vi "Mock Launch Helper Loop.vi"(8 "error in (no error)":errorcluster, 11 "Mock Process in":refnum<class "Mock Process.lvclass">) -> (0 "error out":errorcluster, 3 "Mock Process out":refnum<class "Mock Process.lvclass">)   [LabVIEW 2020, in "Mock Process.lvclass"]
uses:
  Mock Process.lvclass
  C:/Git/astemes-triarc-framework/source/Framework/Helper Loop/Helper Loop.lvclass
  Mock Process.lvclass/Mock Process.ctl
  Framework/Helper Loop/Helper Loop.lvclass
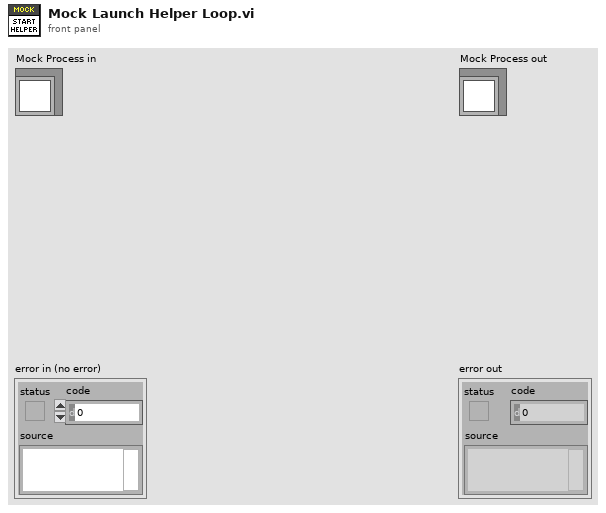
[diagram p1: front panel]
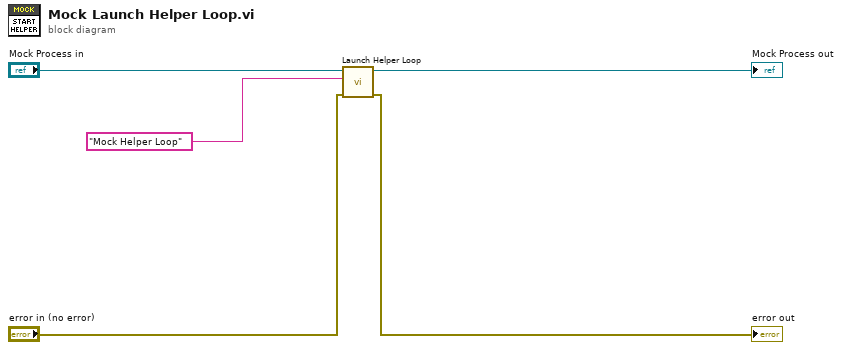
[diagram p0: block diagram]
diagram:
  n1 = call "Launch Helper Loop.vi"("error in (no error)"="error in (no error)", "Message"="Mock Helper Loop", "Helper Loop In"="Mock Process in") -> ("error out"=→"error out":errorcluster, "Helper Loop Out"=→"Mock Process out":refnum<class "Mock Process.lvclass">)  [unwired: 7 in]
